vi "Teleop.vi"(10 "Match Info":T5={"Autonomous Elapsed Seconds"=0.0, "TeleOp Elapsed Seconds"=26.581, "Disabled Elapsed Seconds"=313.725, "Visited Autonomous"=FALSE, "Visited TeleOp"=TRUE, "Visited Disabled"=TRUE, "Autonomous Settings"={"Autonomous Style"=enum."Independent", "VI Refnum"=refnum}}, 11 "Call Context":T6=enum."Stop") -> ()   [LabVIEW 2018]
doc: "This VI is called for each TeleOp packet received from the DS where the robot is not disabled. It is often used to read from the joysticks and update I/O or to update setpoints for timed control loops. It should complete and return within 20 milliseconds or it may miss DS packets."
uses:
  <vilib>/Rock Robotics/WPI/DriverStation/WPI_DriverStationDerivedRobotMode.ctl
  <vilib>/Rock Robotics/WPI/DriverStation/WPI_DriverStationMatch Info.ctl
  <vilib>/Rock Robotics/WPI/ThirdParty/Phoenix-LabVIEW/Motor Controller/Controls/CTRE_Phoenix_MotorControl_ControlMode.ctl
  <vilib>/Rock Robotics/WPI/Utilities/WPI_GetSetVariantRefNum.vi
  <vilib>/Rock Robotics/Network Tables/NT Write Boolean Array.vi
  <vilib>/Rock Robotics/Network Tables/NT Write Numeric Array.vi
  <vilib>/Rock Robotics/WPI/ThirdParty/Phoenix-LabVIEW/Motor Controller/Get/CTRE_Phoenix_MotorController_GetOutputCurrent_Enhanced.vi
  <vilib>/Rock Robotics/WPI/ThirdParty/Phoenix-LabVIEW/Motor Controller/Get/CTRE_Phoenix_MotorController_GetSelectedSensorData.vi
  <vilib>/Rock Robotics/WPI/ThirdParty/Phoenix-LabVIEW/Motor Controller/Get/CTRE_Phoenix_MotorController_GetClosedLoopData.vi
panel:
  out "Velocity":T1(graph)={"Position (Raw Sensor Units)"=4039, "Position (Raw Sensor Units)"=37}
  in  "Continuous Current Limit (Amps)":i32
  in  "Peak Current (Amps)":i32
  in  "Enable Current Limit?":bool
  out "Position":T1(graph)={"Position (Raw Sensor Units)"=4039, "Position (Raw Sensor Units)"=37}
  in  "INvert Left":bool
  in  "Invert Right":bool=TRUE
  in  "Right Sensor Phase":bool=TRUE
  in  "Left Sensor Phase":bool=TRUE
  out "Error":T2(graph)={"Closed-loop Error"=57, "Closed-loop Error"=-37}
  out "Current":T3(graph)={"Output Current"=0.125, "Output Current"=0.25}
  in  "Mode":T4(tab)=enum."NewPID/0Encoders"
  in  "RightSetPosition":dbl
  in  "LeftSetPosition":dbl=4096.0
  in  "Right Set Position":dbl
  in  "Left Set Position":dbl=20000.0
  in  "Max Acceleration":dbl=750.0
  in  "Cruise Velocity":dbl=3500.0
  in  "Zero Encoders":bool=TRUE
  in  "LP":dbl=2.0
  in  "LI":dbl
  in  "LD":dbl=700.0
  in  "LF":dbl
  in  "LI Zone":dbl
  in  "secondsFromNeutralToFull":dbl=0.2
  in  "RP":dbl=3.0
  in  "RI":dbl
  in  "RD":dbl=450.0
  in  "RF":dbl
  in  "allowableClosedLoopError":i32=100
  in  "RI Zone":dbl
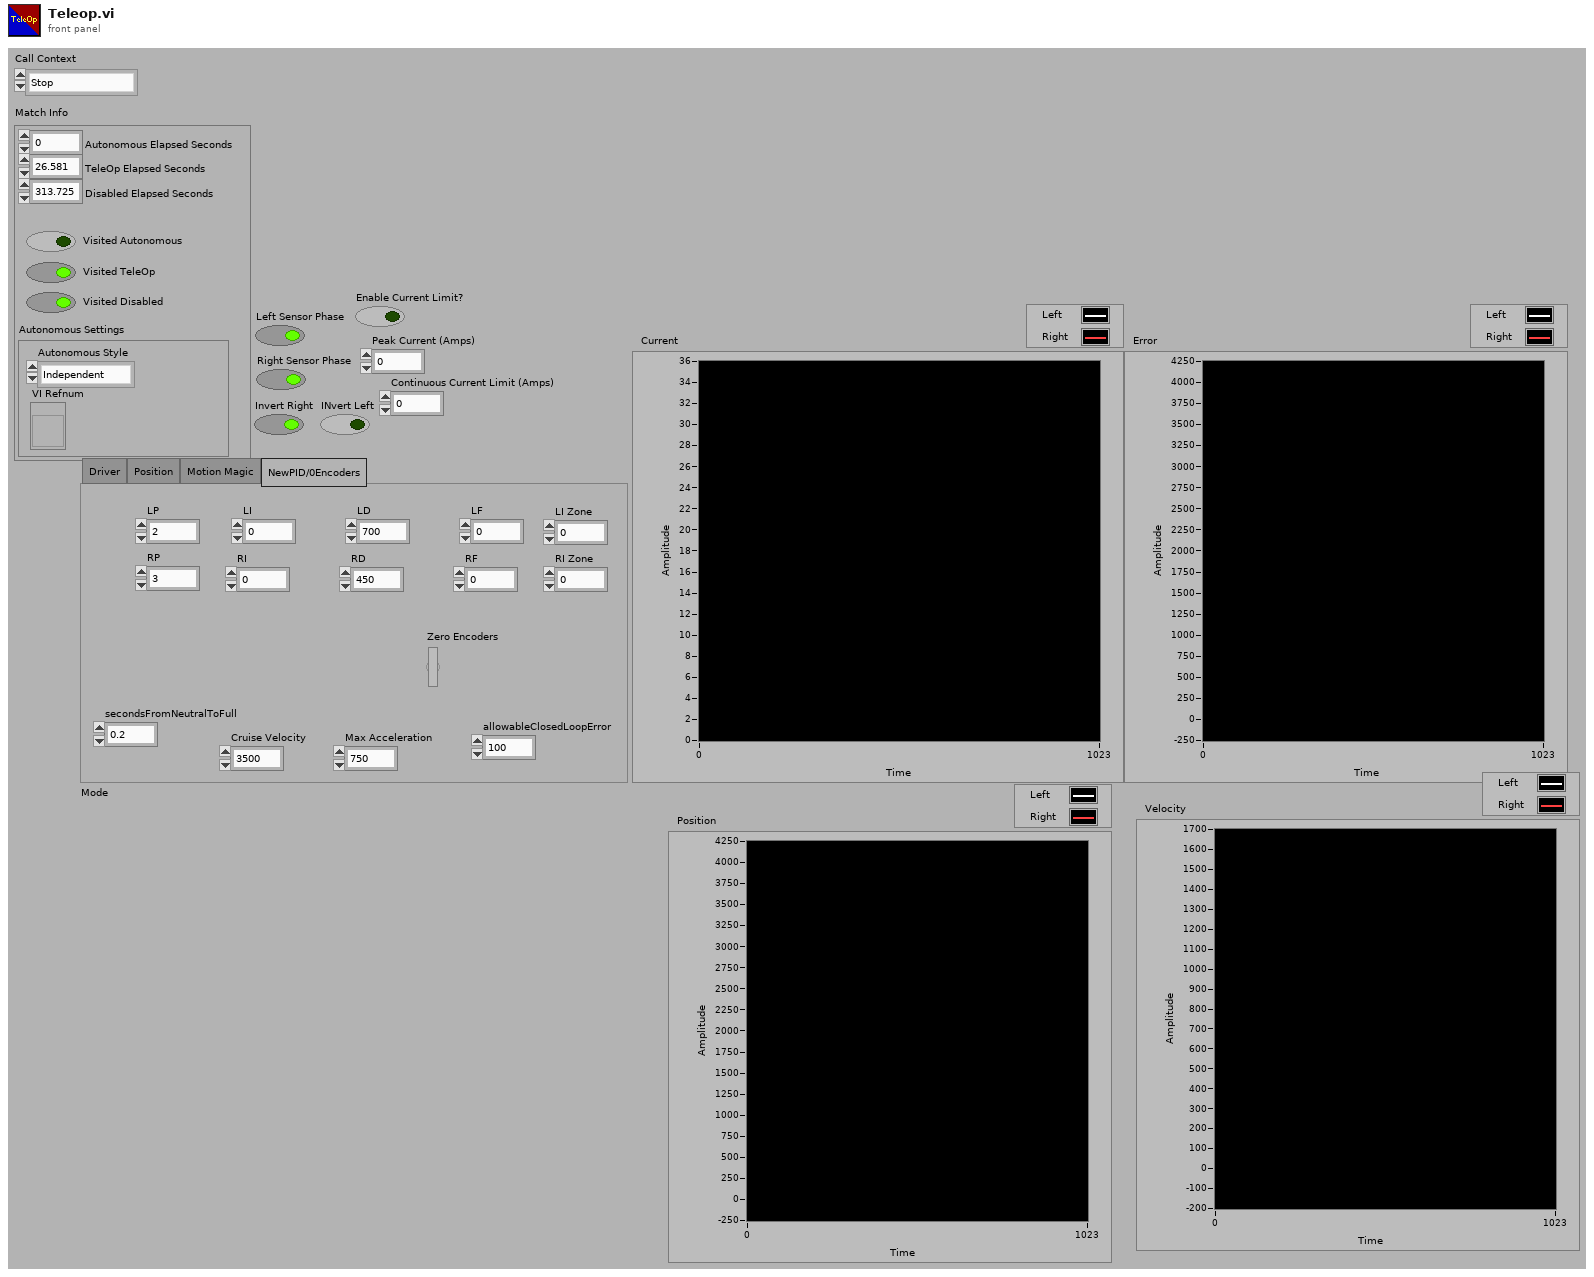
[diagram p1: front panel]
types:
  T1 = cluster{"Position (Raw Sensor Units)":i32, "Position (Raw Sensor Units)":i32}
  T2 = cluster{"Closed-loop Error":i32, "Closed-loop Error":i32}
  T3 = cluster{"Output Current":dbl, "Output Current":dbl}
  T4 = enum32{"Driver", "Position", "Motion Magic", "NewPID/0Encoders"}
  T5 = typedef "WPI_DriverStationMatch Info.ctl" = cluster{"Autonomous Elapsed Seconds":dbl, "TeleOp Elapsed Seconds":dbl, "Disabled Elapsed Seconds":dbl, "Visited Autonomous":bool, "Visited TeleOp":bool, "Visited Disabled":bool, "Autonomous Settings":cluster{"Autonomous Style":enum16{"Iterative", "Independent"}, "VI Refnum":refnum<vi>}}
  T6 = typedef "WPI_DriverStationDerivedRobotMode.ctl" = enum16{"Init", "Execute", "Stop"}
  T7 = typedef "WPI_MotorControlDeviceRef.ctl" = cluster{"DeviceStatus":errorcluster, "Type":T8, "PWM":cluster{"PWM Channel":T9, "DeadBand":T10}, "CAN":cluster{"Device Number":u8, "SetOutput VI Ref":variant, "GetOutput VI Ref":variant, "Enable VI Ref":variant, "Disable VI Ref":variant, "Data":variant}, "Invert":bool, "DIO PWM":cluster{"PWM \"Enable\" Channel":T9, "DIOChannel":T11, "PWM Rate":dbl}}
  T8 = typedef "WPI_MotorControlType.ctl" = enum16{"PWM", "CAN", "DIO PWM"}
  T9 = typedef "FPGA_DIOPWMChannel.ctl" = enum8{"PWM 0", "PWM 1", "PWM 2", "PWM 3", "PWM 4", "PWM 5", "PWM 6", "PWM 7", "PWM 8", "PWM 9", "PWM MXP 0", "PWM MXP 1", "PWM MXP 2", "PWM MXP 3", "PWM MXP 4", "PWM MXP 5", "PWM MXP 6", "PWM MXP 7", "PWM MXP 8", "PWM MXP 9", "Invalid"}
  T10 = typedef "WPI_PWMDeadband.ctl" = cluster{"Name":string, "maxPositivePwm":i32, "minPositivePwm":i32, "centerPwm":i32, "maxNegativePwm":i32, "minNegativePwm":i32, "angularRange":u16}
  T11 = typedef "FPGA_DIOChannel.ctl" = enum8{"DIO 0", "DIO 1", "DIO 2", "DIO 3", "DIO 4", "DIO 5", "DIO 6", "DIO 7", "DIO 8", "DIO 9", "DIO MXP 0", "DIO MXP 1", "DIO MXP 2", "DIO MXP 3", "DIO MXP 4", "DIO MXP 5", "DIO MXP 6", "DIO MXP 7", "DIO MXP 8", "DIO MXP 9", "DIO MXP 10", "DIO MXP 11", "DIO MXP 12", "DIO MXP 13", "DIO MXP 14", "DIO MXP 15", "SPI Port CS1", "SPI Port CS2", "SPI Port CS3", "SPI Port MISO", "SPI Port MOSI", "Invalid"}
  T12 = typedef "CTRE_Phoenix_MotorControl_ControlMode.ctl" = u16
  T13 = typedef "WPI_JoystickDevRef.ctl" = cluster{"Device":T14}
  T14 = typedef "WPI_JoystickDeviceEnum.ctl" = enum16{"USB 0", "USB 1", "USB 2", "USB 3", "USB 4", "USB 5"}
  T15 = cluster{"Velocity (Raw Sensor Units per 100 ms)":i32, "Velocity (Raw Sensor Units per 100 ms)":i32}
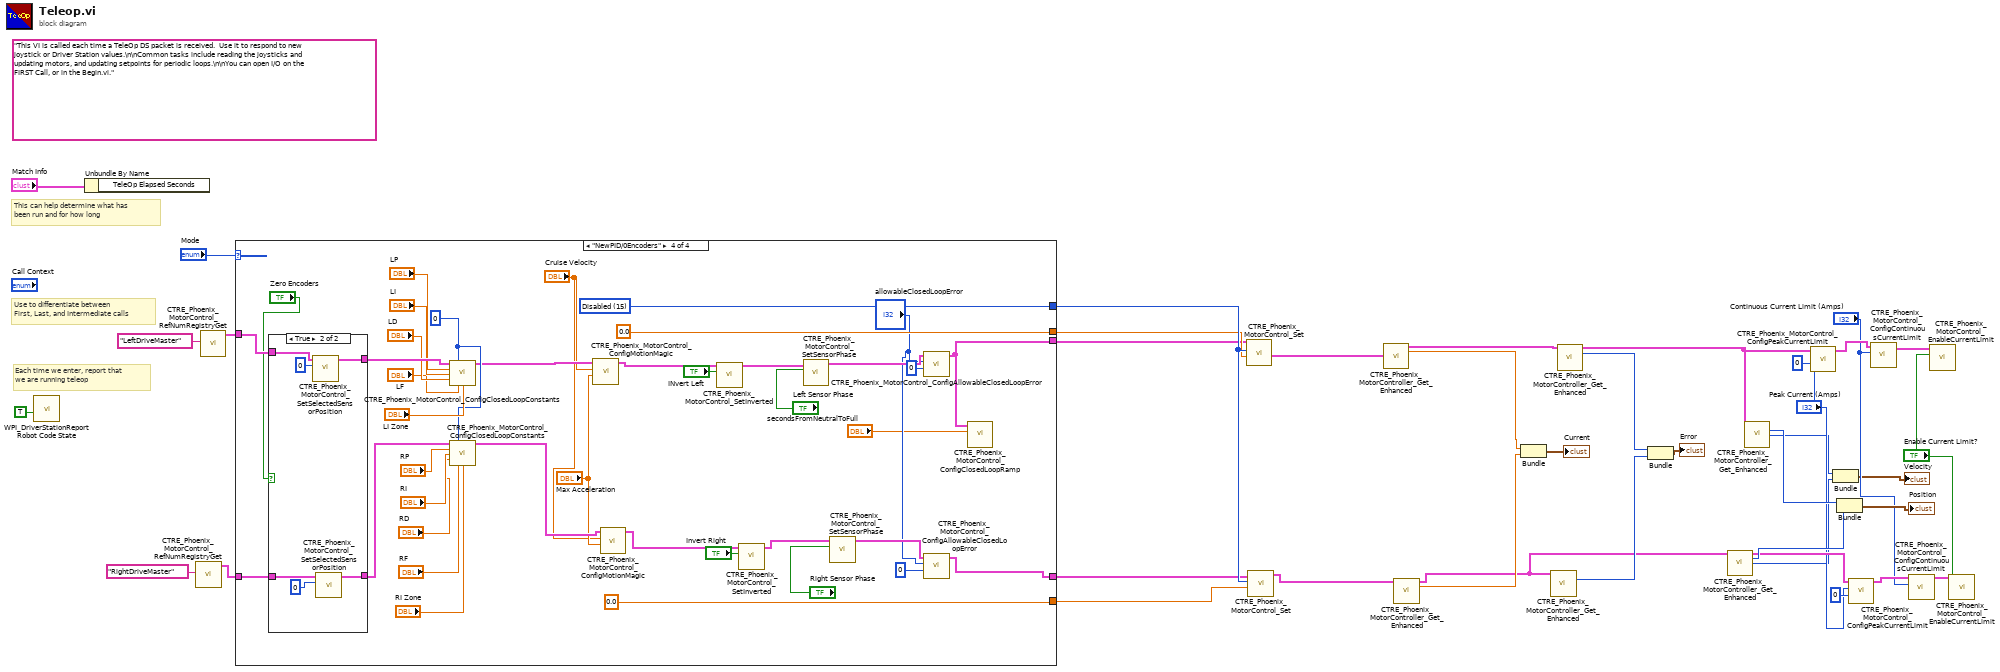
[diagram p0: block diagram]
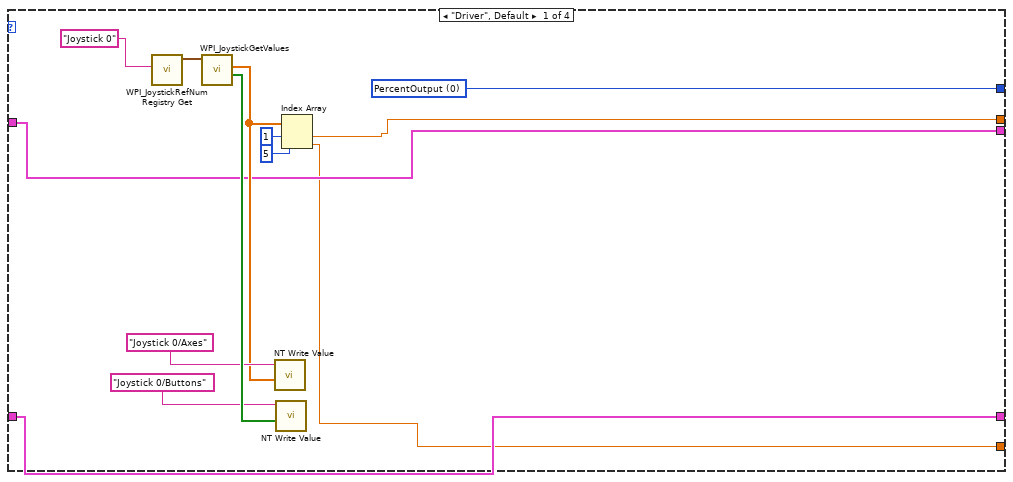
[diagram p2: hidden frame]
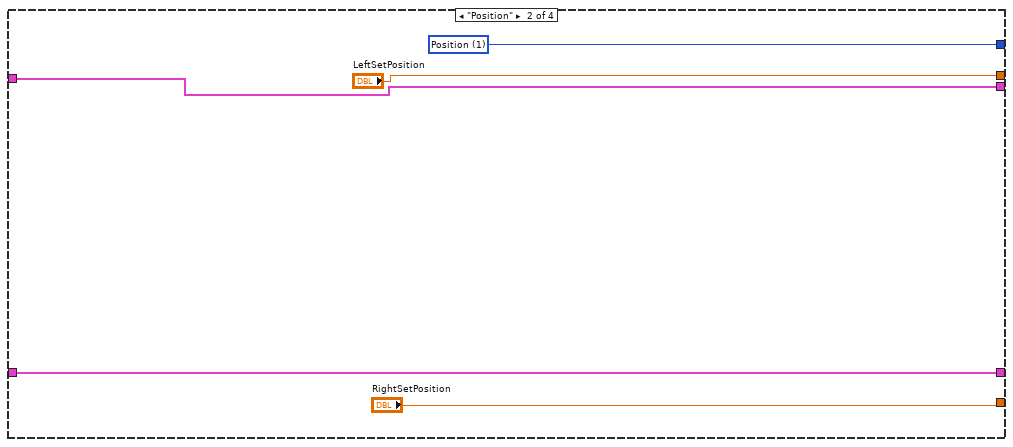
[diagram p3: hidden frame]
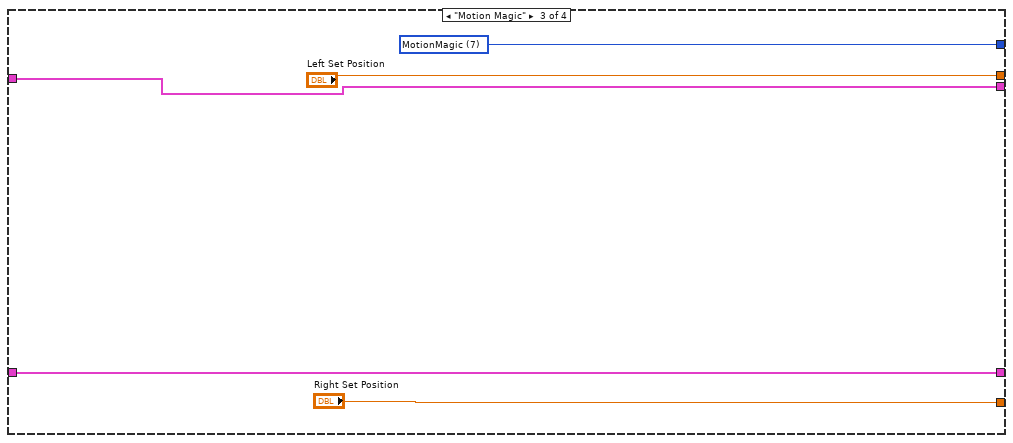
[diagram p4: hidden frame]
diagram:
  (unwired) "This VI is called each time a TeleOp DS packet is received.  Use it to respond to new joystick or Driver Station values.\n\nCommon tasks include reading the joysticks and updating motors, and updating setpoints for periodic loops.\n\nYou can open I/O on the FIRST Call, or in the Begin.vi."
  # "Each time we enter, report that\nwe are running teleop"
  # "Use to differentiate between\nFirst, Last, and Intermediate calls"
  # "This can help determine what has\nbeen run and for how long"
  n1 = call <vilib>:"WPI_DriverStationReport Robot Code State.vi"("TeleOp"=TRUE ("Autonomous")) -> ()  [unwired: 10 in, 1 out]
  n2 = Unbundle By Name("Match Info") -> ()  [unwired: 1 out]
  n3 = call <vilib>:"CTRE_Phoenix_MotorControl_RefNumRegistryGet.vi"("refnum name"="RightDriveMaster") -> ("PhoenixMotorControlDevRef"=w31:T7)  [unwired: 9 in, 1 out]
  n4 = call <vilib>:"CTRE_Phoenix_MotorControl_RefNumRegistryGet.vi"("refnum name"="LeftDriveMaster") -> ("PhoenixMotorControlDevRef"=w29:T7)  [unwired: 9 in, 1 out]
  n5 = case shown="\"NewPID/0Encoders\"" "Mode" {
    tunnel: [w47 w57 w62 w99] -> w36
    tunnel: [w40 "LeftSetPosition" "Left Set Position" 0.0 ("Left Set Position")] -> w35
    tunnel: [w41 "RightSetPosition" "Right Set Position" 0.0 ("Left Set Position")] -> w34
    tunnel: w31 -> [w42 w53 w58 w101]
    tunnel: [w42 w53 w58 w74] -> w30
    tunnel: w29 -> [w43 w54 w59 w100]
    tunnel: [w43 w54 w59 w69] -> w28
    frame "Driver", Default {
      w47 = T12 0 items=["PercentOutput"=0, "Position"=1, "Velocity"=2, "Current"=3, "Follower"=5, "MotionProfile"=6, "MotionMagic"=7, "MotionProfileArc"=10, "Disabled"=15] ("Control Mode")
      n6 = call <vilib>:"WPI_JoystickRefNum Registry Get.vi"("refnum name"="Joystick 0") -> ("JoystickDevRef"=w51:T13)  [unwired: 1 in, 9 out]
      n7 = call <vilib>:"WPI_JoystickGetValues.vi"("JoystickDevRef"=w51) -> ("Buttons"=w52:bool[], "Axes"=w46:dbl[])  [unwired: 6 in, 3 out]
      n8 = call-poly <vilib>:"NT Write Value.vi"("Numeric Array"=w46, "Name"="Joystick 0/Axes") -> ()  [unwired: 9 in, 1 out]
      n9 = call-poly <vilib>:"NT Write Value.vi"("Boolean Array"=w52, "Name"="Joystick 0/Buttons") -> ()  [unwired: 9 in, 1 out]
      n10 = Index Array(array=w46, index #1=1 ("index"), index #2=5 ("index")) -> (element #1=w40:dbl, element #2=w41:dbl)
    }
    frame "Position" {
      w57 = T12 1 items=["PercentOutput"=0, "Position"=1, "Velocity"=2, "Current"=3, "Follower"=5, "MotionProfile"=6, "MotionMagic"=7, "MotionProfileArc"=10, "Disabled"=15] ("Control Mode")
    }
    frame "Motion Magic" {
      w62 = T12 7 items=["PercentOutput"=0, "Position"=1, "Velocity"=2, "Current"=3, "Follower"=5, "MotionProfile"=6, "MotionMagic"=7, "MotionProfileArc"=10, "Disabled"=15] ("Control Mode")
    }
    frame "NewPID/0Encoders" {
      w90 = 0 ("slotIdx")
      w99 = T12 15 items=["PercentOutput"=0, "Position"=1, "Velocity"=2, "Current"=3, "Follower"=5, "MotionProfile"=6, "MotionMagic"=7, "MotionProfileArc"=10, "Disabled"=15] ("Control Mode")
      n11 = case shown="True" "Zero Encoders" {
        tunnel: w101 -> [w102 w107]
        tunnel: w100 -> [w103 w106]
        tunnel: [w103 w105] -> w96
        tunnel: [w102 w104] -> w86
        frame False {
        }
        frame True {
          n12 = call <vilib>:"CTRE_Phoenix_MotorControl_SetSelectedSensorPosition.vi"("New Sensor Position"=0, "PhoenixMotorControlDevRef"=w106) -> ("PhoenixMotorControlDevRef"=w105:T7)  [unwired: 8 in, 1 out]
          n13 = call <vilib>:"CTRE_Phoenix_MotorControl_SetSelectedSensorPosition.vi"("New Sensor Position"=0, "PhoenixMotorControlDevRef"=w107) -> ("PhoenixMotorControlDevRef"=w104:T7)  [unwired: 8 in, 1 out]
        }
      }
      n14 = call <vilib>:"CTRE_Phoenix_MotorControl_ConfigClosedLoopConstants.vi"("PhoenixMotorControlDevRef"=w96, "slotIdx"=w90, "P"="LP", "I"="LI", "D"="LD", "F"="LF", "I Zone"="LI Zone") -> ("PhoenixMotorControlDevRef"=w88:T7)  [unwired: 7 in, 1 out]
      n15 = call <vilib>:"CTRE_Phoenix_MotorControl_ConfigClosedLoopConstants.vi"("PhoenixMotorControlDevRef"=w86, "slotIdx"=w90, "P"="RP", "I"="RI", "D"="RD", "F"="RF", "I Zone"="RI Zone") -> ("PhoenixMotorControlDevRef"=w87:T7)  [unwired: 7 in, 1 out]
      n16 = call <vilib>:"CTRE_Phoenix_MotorControl_ConfigMotionMagic.vi"("Acceleration"="Max Acceleration", "Cruise Velocity"="Cruise Velocity", "PhoenixMotorControlDevRef"=w88) -> ("PhoenixMotorControlDevRef"=w81:T7)  [unwired: 7 in, 1 out]
      n17 = call <vilib>:"CTRE_Phoenix_MotorControl_ConfigMotionMagic.vi"("Acceleration"="Max Acceleration", "Cruise Velocity"="Cruise Velocity", "PhoenixMotorControlDevRef"=w87) -> ("PhoenixMotorControlDevRef"=w79:T7)  [unwired: 7 in, 1 out]
      n18 = call <vilib>:"CTRE_Phoenix_MotorControl_SetInverted.vi"("Invert?"="INvert Left", "PhoenixMotorControlDevRef"=w81) -> ("PhoenixMotorControlDevRef"=w80:T7)  [unwired: 8 in, 1 out]
      n19 = call <vilib>:"CTRE_Phoenix_MotorControl_SetInverted.vi"("Invert?"="Invert Right", "PhoenixMotorControlDevRef"=w79) -> ("PhoenixMotorControlDevRef"=w78:T7)  [unwired: 8 in, 1 out]
      n20 = call <vilib>:"CTRE_Phoenix_MotorControl_SetSensorPhase.vi"("PhaseSensor"="Left Sensor Phase", "PhoenixMotorControlDevRef"=w80) -> ("PhoenixMotorControlDevRef"=w75:T7)  [unwired: 8 in, 1 out]
      n21 = call <vilib>:"CTRE_Phoenix_MotorControl_SetSensorPhase.vi"("PhaseSensor"="Right Sensor Phase", "PhoenixMotorControlDevRef"=w78) -> ("PhoenixMotorControlDevRef"=w73:T7)  [unwired: 8 in, 1 out]
      n22 = call <vilib>:"CTRE_Phoenix_MotorControl_ConfigAllowableClosedLoopError.vi"("slotIdx"=u32 0, "allowableClosedLoopError"="allowableClosedLoopError", "PhoenixMotorControlDevRef"=w75) -> ("PhoenixMotorControlDevRef"=w69:T7)  [unwired: 7 in, 1 out]
      n23 = call <vilib>:"CTRE_Phoenix_MotorControl_ConfigAllowableClosedLoopError.vi"("slotIdx"=u32 0, "allowableClosedLoopError"="allowableClosedLoopError", "PhoenixMotorControlDevRef"=w73) -> ("PhoenixMotorControlDevRef"=w74:T7)  [unwired: 7 in, 1 out]
      n24 = call <vilib>:"CTRE_Phoenix_MotorControl_ConfigClosedLoopRamp.vi"("secondsFromNeutralToFull"="secondsFromNeutralToFull", "PhoenixMotorControlDevRef"=w69) -> ()  [unwired: 8 in, 2 out]
    }
  }
  n25 = call <vilib>:"CTRE_Phoenix_MotorControl_Set.vi"("Output"=w35, "Control Mode"=w36, "PhoenixMotorControlDevRef"=w28) -> ("PhoenixMotorControlDevRef"=w27:T7)  [unwired: 7 in, 1 out]
  n26 = call <vilib>:"CTRE_Phoenix_MotorControl_Set.vi"("Output"=w34, "Control Mode"=w36, "PhoenixMotorControlDevRef"=w30) -> ("PhoenixMotorControlDevRef"=w26:T7)  [unwired: 7 in, 1 out]
  n27 = call-poly <vilib>:"CTRE_Phoenix_MotorController_Get_Enhanced.vi"("PhoenixMotorControlDevRef"=w27) -> ("PhoenixMotorControlDevRef"=w21:T7, "Output Current"=w24:dbl)  [unwired: 12 in, 1 out]
  n28 = call-poly <vilib>:"CTRE_Phoenix_MotorController_Get_Enhanced.vi"("PhoenixMotorControlDevRef"=w26) -> ("PhoenixMotorControlDevRef"=w17:T7, "Output Current"=w23:dbl)  [unwired: 12 in, 1 out]
  n29 = Bundle("Output Current"=w24, "Output Current"=w23) -> (→"Current":T3)  [unwired: 1 in]
  n30 = call-poly <vilib>:"CTRE_Phoenix_MotorController_Get_Enhanced.vi"("PhoenixMotorControlDevRef"=w17) -> ("Closed-loop Error"=w20:i32)  [unwired: 9 in, 5 out]
  n31 = call-poly <vilib>:"CTRE_Phoenix_MotorController_Get_Enhanced.vi"("PhoenixMotorControlDevRef"=w21) -> ("PhoenixMotorControlDevRef"=w10:T7, "Closed-loop Error"=w15:i32)  [unwired: 9 in, 4 out]
  n32 = Bundle("Closed-loop Error"=w15, "Closed-loop Error"=w20) -> (→"Error":T2)  [unwired: 1 in]
  n33 = call-poly <vilib>:"CTRE_Phoenix_MotorController_Get_Enhanced.vi"("PhoenixMotorControlDevRef"=w17) -> ("PhoenixMotorControlDevRef"=w14:T7, "Position (Raw Sensor Units)"=w18:i32, "Velocity (Raw Sensor Units per 100 ms)"=w1:i32)  [unwired: 11 in, 1 out]
  n34 = call-poly <vilib>:"CTRE_Phoenix_MotorController_Get_Enhanced.vi"("PhoenixMotorControlDevRef"=w10) -> ("Position (Raw Sensor Units)"=w19:i32, "Velocity (Raw Sensor Units per 100 ms)"=w2:i32)  [unwired: 11 in, 2 out]
  n35 = call <vilib>:"CTRE_Phoenix_MotorControl_ConfigPeakCurrentLimit.vi"("Peak Current Maximum Duration (ms)"=0, "Peak Current (Amps)"="Peak Current (Amps)", "PhoenixMotorControlDevRef"=w10) -> ("PhoenixMotorControlDevRef"=w9:T7)  [unwired: 7 in, 1 out]
  n36 = Bundle("Velocity (Raw Sensor Units per 100 ms)"=w2, "Velocity (Raw Sensor Units per 100 ms)"=w1) -> (→"Velocity":T15)  [unwired: 1 in]
  n37 = Bundle("Position (Raw Sensor Units)"=w19, "Position (Raw Sensor Units)"=w18) -> (→"Position":T1)  [unwired: 1 in]
  n38 = call <vilib>:"CTRE_Phoenix_MotorControl_ConfigPeakCurrentLimit.vi"("Peak Current Maximum Duration (ms)"=0, "Peak Current (Amps)"="Peak Current (Amps)", "PhoenixMotorControlDevRef"=w14) -> ("PhoenixMotorControlDevRef"=w12:T7)  [unwired: 7 in, 1 out]
  n39 = call <vilib>:"CTRE_Phoenix_MotorControl_ConfigContinuousCurrentLimit.vi"("Continuous Current Limit (Amps)"="Continuous Current Limit (Amps)", "PhoenixMotorControlDevRef"=w9) -> ("PhoenixMotorControlDevRef"=w8:T7)  [unwired: 8 in, 1 out]
  n40 = call <vilib>:"CTRE_Phoenix_MotorControl_ConfigContinuousCurrentLimit.vi"("Continuous Current Limit (Amps)"="Continuous Current Limit (Amps)", "PhoenixMotorControlDevRef"=w12) -> ("PhoenixMotorControlDevRef"=w7:T7)  [unwired: 8 in, 1 out]
  n41 = call <vilib>:"CTRE_Phoenix_MotorControl_EnableCurrentLimit.vi"("Enable Current Limit?"="Enable Current Limit?", "PhoenixMotorControlDevRef"=w8) -> ()  [unwired: 8 in, 2 out]
  n42 = call <vilib>:"CTRE_Phoenix_MotorControl_EnableCurrentLimit.vi"("Enable Current Limit?"="Enable Current Limit?", "PhoenixMotorControlDevRef"=w7) -> ()  [unwired: 8 in, 2 out]
